vi "Window-Exit confirmation.vi"() -> (0 "error out":errorcluster, 2 "Cancelled":bool)   [LabVIEW 2013]
doc: "Use this template to create a dialog box with event handling."
uses:
  <vilib>/Utility/miscctls.llb/LVPointTypeDef.ctl
  Global Variables/General Globals.vi
panel:
  in  "Cancel":bool
  in  "OK":bool
  # "Are you sure you want to close the viewer's window?"
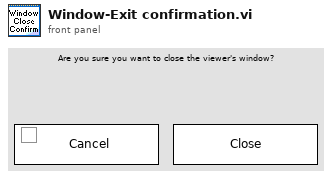
[diagram p1: front panel]
types:
  T1 = typedef "LVPointTypeDef.ctl" = cluster{"Horizontal":i16, "Vertical":i16}
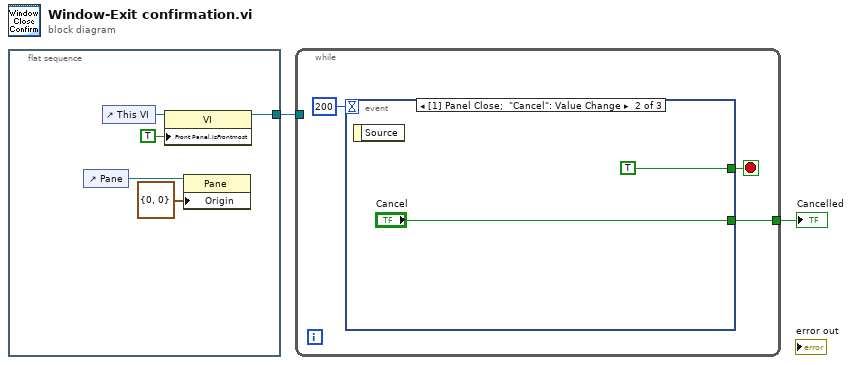
[diagram p0: block diagram]
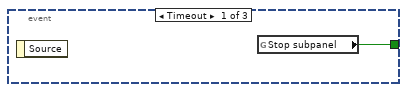
[diagram p2: hidden frame]
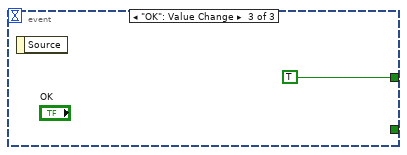
[diagram p3: hidden frame]
diagram:
  n1 = flat-sequence {
    tunnel: [w5] -> w2
    frame #0 {
      n2 = control-ref of="Pane"() -> (w3:refnum<vi>)
      n3 = control-ref of="This VI"() -> (w6:refnum<vi>)
      n4 = property on="Property Node" class="VI"(reference=w6, "Front Panel.IsFrontmost"=TRUE ("Front Panel Window:Is Frontmost")) -> (reference out=w5:refnum<vi>)  [unwired: 1 in, 1 out]
      n5 = property class="Pane"(reference=w3, "Origin"=T1 {"Horizontal"=0, "Vertical"=0}) -> ()  [unwired: 1 in, 2 out]
    }
  }
  n6 = while {
    tunnel: w2 -> [_]
    tunnel: [w8] -> w1
    stop <- w10 stop-if-true
    n7 = event shown="[1] Panel Close;  \"Cancel\": Value Change" {
      selector: _ -> [_ _ _]
      dyn-events: _ -> [_ _ _]
      timeout: 200 -> [_ _ _]
      tunnel: [w11 TRUE ("Stop?") TRUE ("Stop?")] -> w10
      tunnel: [_ "Cancel" _] -> w8
      event Timeout {
        n8 = event-data() -> ()  [unwired: 1 in, 1 out]
        n9 = global read "General Globals.vi" "Stop subpanel"() -> (w11:bool)
      }
      event Panel Close; "Cancel": Value Change {
        n10 = event-data() -> ()  [unwired: 1 in, 1 out]
      }
      event "OK": Value Change {
        n11 = event-data() -> ()  [unwired: 1 in, 1 out]
      }
    }
  }
  "Cancelled" <- w1
